vi "Channel_ToClass.vi"(8 "error in (no error)":errorcluster, 11 "Item Ref in":T1 format="%.0x") -> (0 "error out":errorcluster, 2 "Wfm?":bool, 3 "Channel out":refnum<class "Channel.lvclass">)   [LabVIEW 2024, in "Embedded TDMS Logger System Explorer.lvlib"]
doc: "Creates a channel class from the VeriStand System Definition File Custom Device channel defined by the item ref in."
uses:
  Embedded TDMS Logger System Explorer.lvlib
  <vilib>/NI VeriStand/Custom Device API/Custom Device Item Ref.ctl
  Shared/File Classes/Channel/Channel.lvclass
  Shared/File Classes/Meta Data.ctl
  <vilib>/NI VeriStand/Custom Device API/Get Item Property (I32).vi
  <vilib>/NI VeriStand/Custom Device API/Get Item Property (Boolean).vi
  <vilib>/NI VeriStand/Custom Device API/Get Item Property (Variant).vi
  <vilib>/NI VeriStand/Custom Device API/Get Item Property (Dependent Node Pointer).vi
  <vilib>/NI VeriStand/Custom Device API/Custom Device API.lvlib
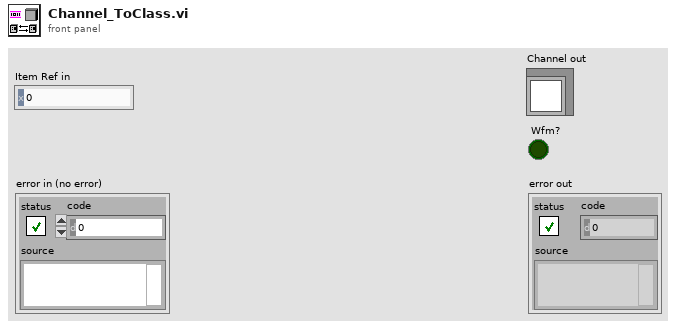
[diagram p1: front panel]
types:
  T1 = typedef "Custom Device API.lvlib/Custom Device Item Ref.ctl" = u64
  T2 = typedef "Meta Data.ctl" = cluster{"Key":string, "Value":string}
  T3 = typedef "Custom Device API.lvlib/Custom Device Item Info.ctl" = cluster{"Name":string, "Is Channel":bool, "GUID":string, "Is Waveform":bool}
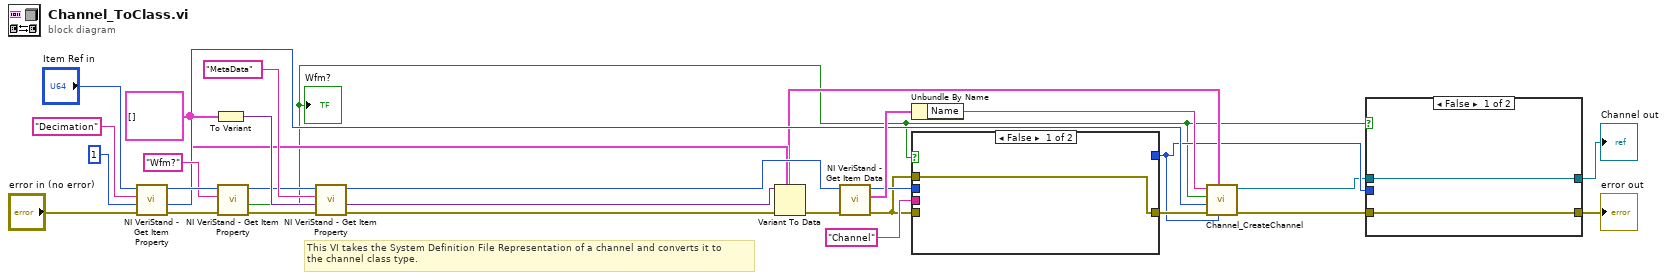
[diagram p0: block diagram]
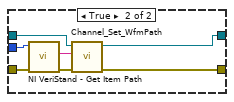
[diagram p2: hidden frame]
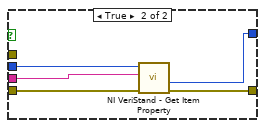
[diagram p3: hidden frame]
diagram:
  w14 = T2[] []
  # "This VI takes the System Definition File Representation of a channel and converts it to\nthe channel class type."
  n1 = call-poly <vilib>:"NI VeriStand - Get Item Property.vi"("error in (no error)"="error in (no error)", "Default Value"=1, "Property Name"="Decimation", "Item Ref in"="Item Ref in") -> ("error out"=w22:errorcluster, "Value"=w15:i32, "Item Ref out"=w27:T1)  [unwired: 4 in, 1 out]
  n2 = To Variant(anything=w14) -> (Variant=w25:variant)
  n3 = call-poly <vilib>:"NI VeriStand - Get Item Property.vi"("error in (no error)"=w22, "Property Name"="Wfm?", "Item Ref in"=w27) -> ("error out"=w21:errorcluster, "Value"=w2:bool, "Item Ref out"=w24:T1)  [unwired: 5 in, 1 out]
  "Wfm?" <- w2
  n4 = call-poly <vilib>:"NI VeriStand - Get Item Property.vi"("error in (no error)"=w21, "Default Value"=w25, "Property Name"="MetaData", "Item Ref in"=w24) -> ("error out"=w12:errorcluster, "Value"=w13:variant, "Item Ref out"=w23:T1)  [unwired: 4 in, 1 out]
  n5 = Variant To Data(error in=w12, type=w14, Variant=w13) -> (data=w10:T2[], error out=w11:errorcluster)
  n6 = call <vilib>:"NI VeriStand - Get Item Data.vi"("error in (no error)"=w11, "Item Ref in"=w23) -> ("error out"=w1:errorcluster, "Item Info"=w19:T3, "Item Ref out"=w17:T1)  [unwired: 7 out]
  n7 = Unbundle By Name(w19) -> ("Name"=w16:string)
  n8 = case shown="False" w2 {
    tunnel: "Channel" ("Property Name") -> [_ w36]
    tunnel: w17 -> [_ w35]
    tunnel: w1 -> [_ w34]
    tunnel: [w31 w33] -> w9
    tunnel: [_ w32] -> w7
    tunnel: w1 -> [w31 _]
    frame False {
    }
    frame True {
      n9 = call-poly <vilib>:"NI VeriStand - Get Item Property.vi"("error in (no error)"=w34, "Property Name"=w36, "Item Ref in"=w35) -> ("error out"=w33:errorcluster, "Dependent Node Ref"=w32:T1)  [unwired: 5 in, 2 out]
    }
  }
  n10 = call "Channel_CreateChannel.vi"("Data Reference"=w7, "Meta Data"=w10, "error in (no error)"=w9, "Decimation"=w15, "Wfm?"=w2, "Name"=w16) -> ("error out"=w6:errorcluster, "Channel out"=w5:refnum<class "Channel.lvclass">)  [unwired: 4 in]
  n11 = case shown="False" w2 {
    tunnel: w7 -> [_ w45]
    tunnel: w6 -> [w37 w44]
    tunnel: w5 -> [w38 w43]
    tunnel: [w37 w40] -> w4
    tunnel: [w38 w39] -> w3
    frame False {
    }
    frame True {
      n12 = call <vilib>:"NI VeriStand - Get Item Path.vi"("error in (no error)"=w44, "Item Ref in"=w45) -> ("error out"=w41:errorcluster, "Path"=w42:string)  [unwired: 6 in, 2 out]
      n13 = call-dynamic "Channel_Set_WfmPath.vi"("error in (no error)"=w41, "WfmPath"=w42, "Channel in"=w43) -> ("error out"=w40:errorcluster, "Channel out"=w39:refnum<class "Channel.lvclass">)  [unwired: 7 in]
    }
  }
  "Channel out" <- w3
  "error out" <- w4
